vi "Shutdown.vi"(8 "error in (no error)":errorcluster, 10 "config path":path, 11 "Lamp in":refnum<class "Lamp.lvclass">) -> (0 "error out":errorcluster, 3 "Lamp out":refnum<class "Lamp.lvclass">)   [LabVIEW 2016, in "Lamp.lvclass"]
uses:
  Lamp.lvclass
  <vilib>/Utility/config.llb/Write Key (Double).vi
  <vilib>/Utility/config.llb/NI_LVConfig.lvlib
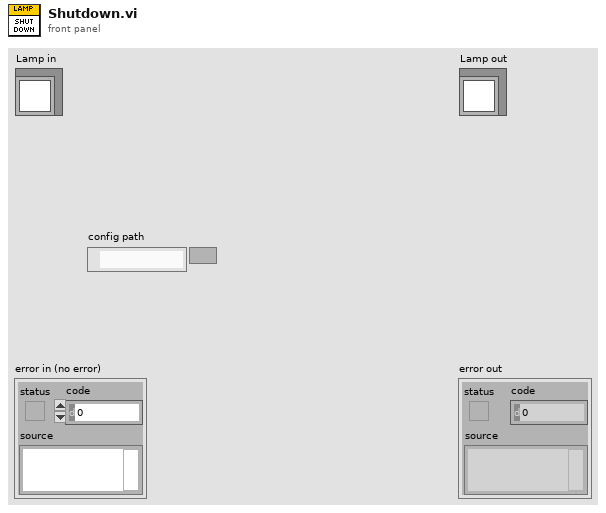
[diagram p1: front panel]
types:
  T1 = typedef "NI_LVConfig.lvlib/Config Data RefNum.ctl" = refnum<k1>
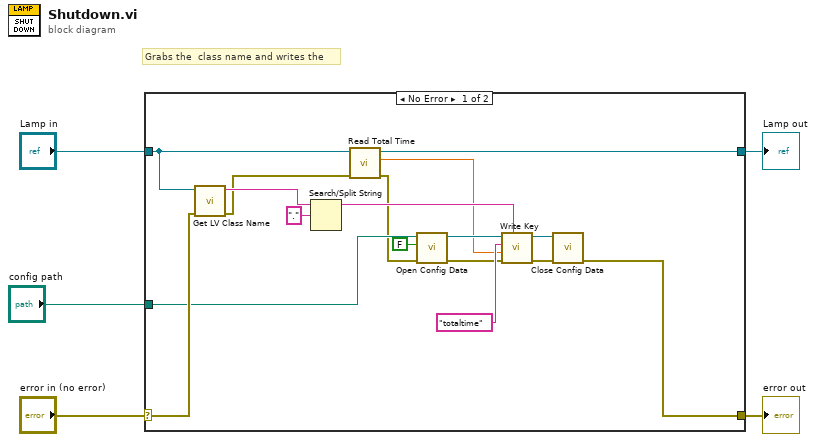
[diagram p0: block diagram]
diagram:
  # "Grabs the  class name and writes the"
  n1 = case shown="No Error" "error in (no error)" {
    selector: "error in (no error)" -> [w22 w24]
    tunnel: [w8 w24] -> w4
    tunnel: [w14 w23] -> w2
    tunnel: "Lamp in" -> [w6 w23]
    tunnel: "config path" -> [w19 _]
    frame No Error {
      n2 = call <vilib>:"Get LV Class Name.vi"("error in (no error)"=w22, "object"=w6) -> ("error out"=w7:errorcluster, "class name"=w21:string)  [unwired: 8 in]
      n3 = Search/Split String(string=w21, search string/char (-)=".") -> (substring before match=w16:string)  [unwired: 1 in, 2 out]
      n4 = call-dynamic "Read Total Time.vi"("error in (no error)"=w7, "Lamp in"=w6) -> ("error out"=w12:errorcluster, "Total Time"=w10:dbl, "Lamp out"=w14:refnum<class "Lamp.lvclass">)  [unwired: 7 in]
      n5 = call <vilib>:"Open Config Data.vi"("error in (no error)"=w12, "create file if necessary (T)"=FALSE, "configuration file path"=w19) -> ("error out"=w11:errorcluster, "refnum"=w17:T1)  [unwired: 6 in, 1 out]
      n6 = call-poly <vilib>:"Write Key.vi"("section"=w16, "error in (no error)"=w11, "value"=w10, "key"="totaltime", "refnum"=w17) -> ("error out"=w9:errorcluster, "refnum out"=w13:T1)  [unwired: 4 in, 1 out]
      n7 = call <vilib>:"Close Config Data.vi"("error in (no error)"=w9, "refnum"=w13) -> ("error out"=w8:errorcluster)  [unwired: 8 in, 1 out]
    }
    frame Error {
    }
  }
  "error out" <- w4
  "Lamp out" <- w2
